vi "AMI1700eth_meas_he_lev.vi"(8 "error in":errorcluster, 11 "conn_id_in":refnum<k5>) -> (0 "error out":errorcluster, 2 "level":dbl, 3 "conn_id_out":refnum<k5>, 4 "status":bool)   [LabVIEW 2019]
panel:
  out "string 2":string
  out "string 1":string
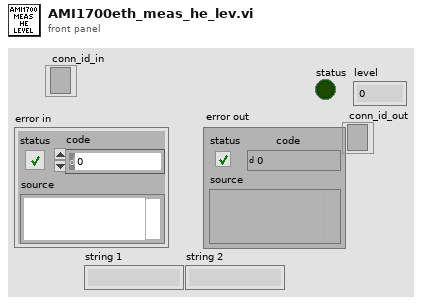
[diagram p1: front panel]
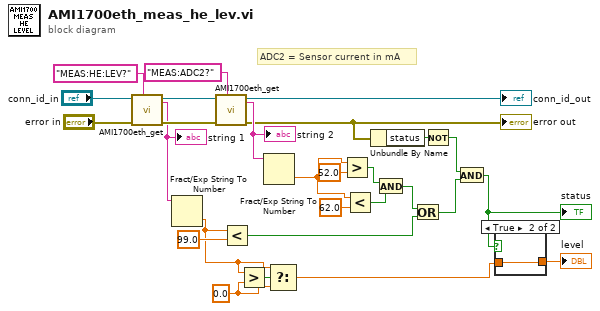
[diagram p0: block diagram]
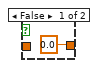
[diagram p2: hidden frame]
diagram:
  w3 = 0.0 ("f")
  # "ADC2 = Sensor current in mA"
  n1 = call "AMI1700eth_get.vi"("command"="MEAS:HE:LEV?" ("string"), "error in"="error in", "conn_id_in"="conn_id_in") -> ("error out"=w25:errorcluster, "conn_id_out"=w26:refnum<k5>, "string"=w17:string)  [unwired: 5 in, 1 out]
  "string 1" <- w17
  n2 = Fract/Exp String To Number(string=w17) -> (number=w2:dbl)  [unwired: 3 in, 1 out]
  n3 = call "AMI1700eth_get.vi"("command"="MEAS:ADC2?" ("string"), "error in"=w25, "conn_id_in"=w26) -> ("error out"=w9:errorcluster, "conn_id_out"=→"conn_id_out":refnum<k5>, "string"=w24:string)  [unwired: 5 in, 1 out]
  "error out" <- w9
  "string 2" <- w24
  n4 = Less?(x=w2, y=99.0) -> (x < y?=w15:bool)
  n5 = Greater?(x=w2, y=w3) -> (0:w4:bool)
  n6 = Fract/Exp String To Number(string=w24) -> (number=w19:dbl)  [unwired: 3 in, 1 out]
  n7 = Select(t=w2, s=w4, f=w3) -> (s? t:f=w1:dbl)
  n8 = Greater?(x=w19, y=52.0) -> (0:w21:bool)
  n9 = Less?(x=w19, y=62.0) -> (x < y?=w20:bool)
  n10 = Unbundle By Name(w9) -> ("status"=w8:bool)
  n11 = And(x=w21, y=w20) -> (x .and. y?=w16:bool)
  n12 = Or(x=w16, y=w15) -> (x .or. y?=w7:bool)
  n13 = Not(x=w8) -> (.not. x?=w6:bool)
  n14 = And(x=w6, y=w7) -> (x .and. y?=w5:bool)
  "status" <- w5
  n15 = case shown="True" w5 {
    tunnel: [0.0 w29] -> w14
    tunnel: w1 -> [_ w29]
    frame False {
    }
    frame True {
    }
  }
  "level" <- w14
